vi "main.vi"() -> ()   [LabVIEW 2017]
uses:
  FaceletColorRing.ctl
  Projekt-Rubik-Library/FaceSymbols.ctl
  <userlib>/RubikSourceLibrary/SingmasterMoves.ctl
panel:
  in  "stop":bool
  in  "Face Symbols":T1
  out "Edge&Corner (Symbols)":string[](array[string])
  out "Corners (Faces,Symbols)":T2[][](array[typedef])
  out "Edges&Corners (Colors)":string[](array[string])
  out "Edges (Faces,Symbols)":T2[][](array[typedef])
  in  "Down Face":T3[][](array[typedef])
  in  "Back Face":T3[][](array[typedef])
  in  "Right Face":T3[][](array[typedef])
  in  "Front Face":T3[][](array[typedef])
  in  "Left Face":T3[][](array[typedef])
  in  "Upper Face":T3[][](array[typedef])
  in  "Check":bool
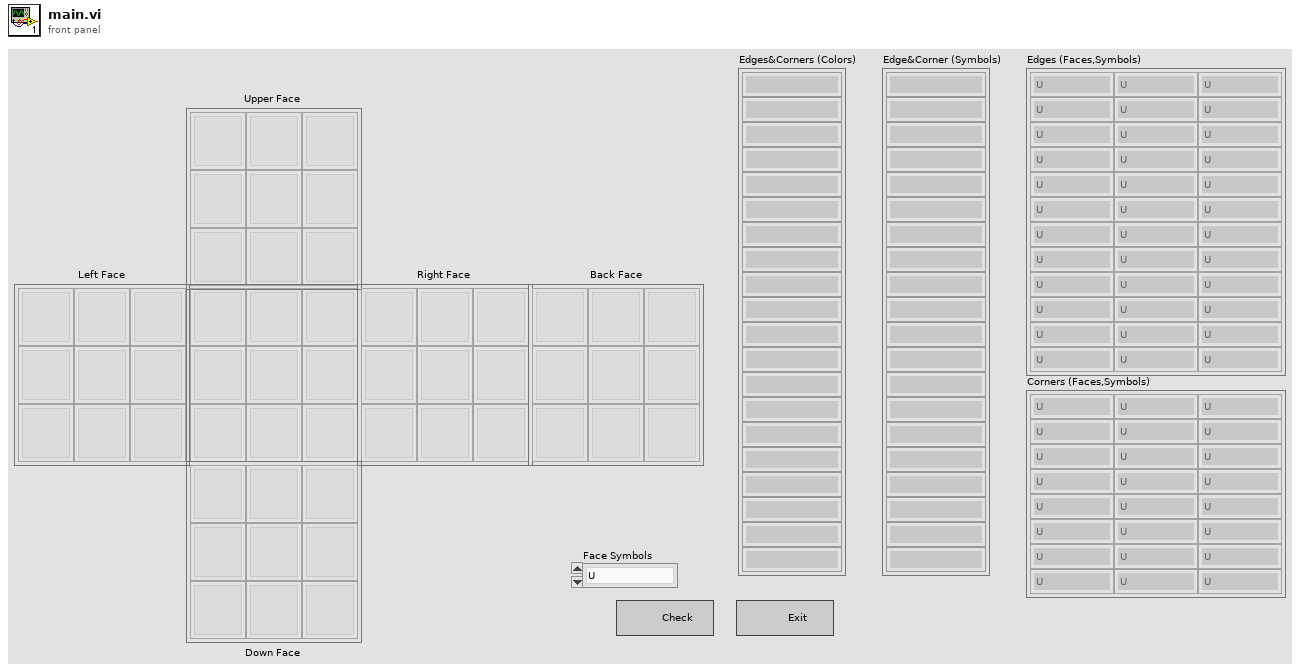
[diagram p1: front panel]
types:
  T1 = typedef "SingmasterMoves.ctl" = enum16{"U", "L", "F", "R", "B", "D"}
  T2 = typedef "FaceSymbols.ctl" = enum16{"U", "L", "F", "R", "B", "D"}
  T3 = typedef "FaceletColorRing.ctl" = u16
  T4 = typedef "FaceletID.ctl" = cluster{i32, i32, "Face Color":T2}
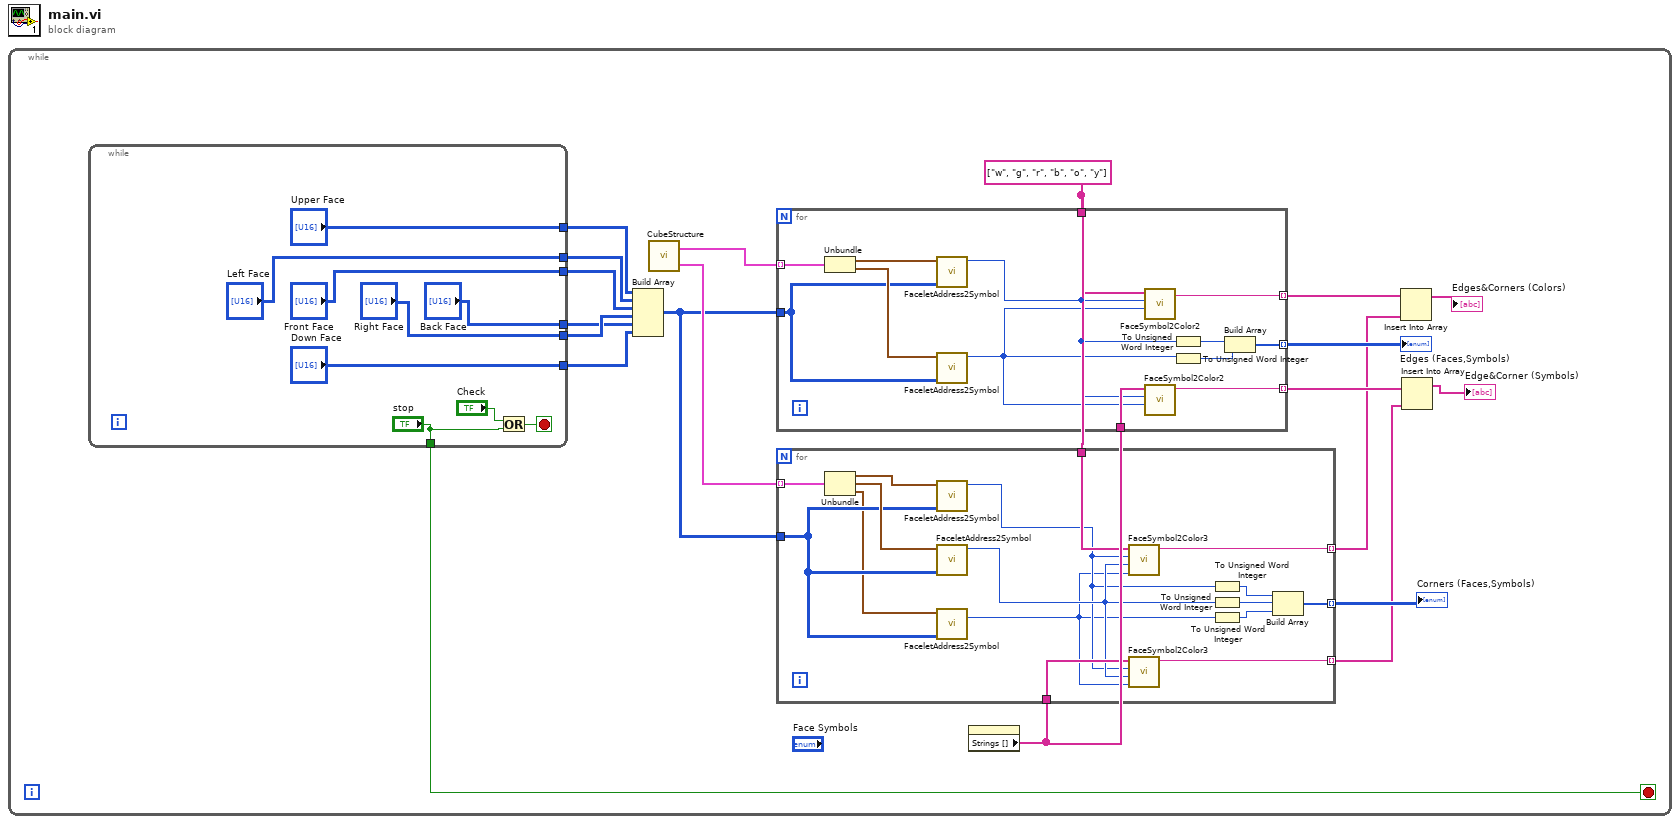
[diagram p0: block diagram]
diagram:
  n1 = while {
    stop <- w1 stop-if-true
    w7 = string[] ["w", "g", "r", "b", "o", "y"]
    n2 = while {
      tunnel: ["Upper Face"] -> w17
      tunnel: ["Left Face"] -> w16
      tunnel: ["Front Face"] -> w15
      tunnel: ["Right Face"] -> w14
      tunnel: ["Back Face"] -> w13
      tunnel: ["Down Face"] -> w12
      tunnel: ["stop"] -> w1
      stop <- w52 stop-if-true
      n3 = Or(x="Check", y="stop") -> (x .or. y?=w52:bool)
    }
    n4 = Build Array(w17, w16, w15, w14, w13, w12) -> (w18:T3[][][])
    n5 = call "CubeStructure.vi"() -> ("cube structure array (8 corners)"=w19:cluster{T4, "element":T4, "element":T4}[], "cube structure array (12 edges)"=w20:cluster{T4, "element":T4}[])  [unwired: 2 in]
    n6 = property on="Face Symbols" class="Enum (strict)"() -> ("Strings []"=w6:string[])  [unwired: 2 in, 2 out]
    n7 = for {
      tunnel: w20 -> [w49] mode=indexing
      tunnel: w18 -> [w38]
      tunnel: w7 -> [w46]
      tunnel: [w47] -> w11 mode=indexing
      tunnel: [w43] -> w9 mode=indexing
      tunnel: w6 -> [w42]
      tunnel: [w40] -> w4 mode=indexing
      n8 = Unbundle(w49) -> (w39:T4, "element"=w48:T4)
      n9 = call "FaceletAddress2Symbol.vi"("Array"=w38, "element"=w39) -> ("Pict Ring"=w37:T3)  [unwired: 9 in]
      n10 = call "FaceletAddress2Symbol.vi"("Array"=w38, "element"=w48) -> ("Pict Ring"=w41:T3)  [unwired: 9 in]
      n11 = call "FaceSymbol2Color2.vi"("Pict Ring"=w41, "Pict Ring 2"=w37, "Array"=w46) -> ("String"=w47:string)  [unwired: 8 in]
      n12 = call "FaceSymbol2Color2.vi"("Pict Ring"=w41, "Pict Ring 2"=w37, "Array"=w42) -> ("String"=w40:string)  [unwired: 8 in]
      n13 = To Unsigned Word Integer(number=w37) -> (unsigned 16bit integer=w45:T3)
      n14 = To Unsigned Word Integer(number=w41) -> (unsigned 16bit integer=w44:T3)
      n15 = Build Array(w45, w44) -> (w43:T3[])
    }
    "Edges (Faces,Symbols)" <- w9
    n16 = for {
      tunnel: w19 -> [w36] mode=indexing
      tunnel: w18 -> [w24]
      tunnel: w7 -> [w29]
      tunnel: [w33] -> w8 mode=indexing
      tunnel: w6 -> [w30]
      tunnel: [w31] -> w3 mode=indexing
      tunnel: [w28] -> w2 mode=indexing
      n17 = Unbundle(w36) -> (w27:T4, "element"=w26:T4, "element"=w23:T4)
      n18 = call "FaceletAddress2Symbol.vi"("Array"=w24, "element"=w27) -> ("Pict Ring"=w22:T3)  [unwired: 9 in]
      n19 = call "FaceletAddress2Symbol.vi"("Array"=w24, "element"=w26) -> ("Pict Ring"=w25:T3)  [unwired: 9 in]
      n20 = call "FaceletAddress2Symbol.vi"("Array"=w24, "element"=w23) -> ("Pict Ring"=w21:T3)  [unwired: 9 in]
      n21 = call "FaceSymbol2Color3.vi"("Pict Ring 3"=w21, "Pict Ring"=w25, "Pict Ring 2"=w22, "Array"=w29) -> ("String"=w28:string)  [unwired: 7 in]
      n22 = call "FaceSymbol2Color3.vi"("Pict Ring 3"=w21, "Pict Ring"=w25, "Pict Ring 2"=w22, "Array"=w30) -> ("String"=w31:string)  [unwired: 7 in]
      n23 = To Unsigned Word Integer(number=w22) -> (unsigned 16bit integer=w32:T3)
      n24 = To Unsigned Word Integer(number=w25) -> (unsigned 16bit integer=w35:T3)
      n25 = To Unsigned Word Integer(number=w21) -> (unsigned 16bit integer=w34:T3)
      n26 = Build Array(w32, w35, w34) -> (w33:T3[])
    }
    "Corners (Faces,Symbols)" <- w8
    n27 = Insert Into Array(array=w11, new element=w2) -> (→"Edges&Corners (Colors)":string[])  [unwired: 1 in]
    n28 = Insert Into Array(array=w4, new element=w3) -> (→"Edge&Corner (Symbols)":string[])  [unwired: 1 in]
  }
